vi "Save info to spreadsheet.vi"(8 "Cell Settings Array":T1(array[cluster])=[{"Cell Position"=1, "Cell Label"="", "Pixel to measure"=0, "Area (cm^2)"=0.126, "Variable"="", "Variable value"="", "Scan settings in queue"=0}, {"Cell Position"=2, "Cell Label"="", "Pixel to measure"=0, "Area (cm^2)"=0.126, "Variable"="", "Variable value"="", "Scan settings in queue"=0}, {"Cell Position"=3, "Cell Label"="", "Pixel to measure"=0, "Area (cm^2)"=0.126, "Variable"="", "Variable value"="", "Scan settings in queue"=0}, {"Cell Position"=4, "Cell Label"="", "Pixel to measure"=0, "Area (cm^2)"=0.126, "Variable"="", "Variable value"="", "Scan settings in queue"=0}, {"Cell Position"=5, "Cell Label"="", "Pixel to measure"=0, "Area (cm^2)"=0.126, "Variable"="", "Variable value"="", "Scan settings in queue"=0}, {"Cell Position"=6, "Cell Label"="", "Pixel to measure"=0, "Area (cm^2)"=0.126, "Variable"="", "Variable value"="", "Scan settings in queue"=0}, {"Cell Position"=7, "Cell Label"="", "Pixel to measure"=0, "Area (cm^2)"=0.126, "Variable"="", "Variable value"="", "Scan settings in queue"=0}, {"Cell Position"=8, "Cell Label"="", "Pixel to measure"=0, "Area (cm^2)"=0.126, "Variable"="", "Variable value"="", "Scan settings in queue"=0}, {"Cell Position"=9, "Cell Label"="", "Pixel to measure"=0, "Area (cm^2)"=0.126, "Variable"="", "Variable value"="", "Scan settings in queue"=0}, {"Cell Position"=10, "Cell Label"="", "Pixel to measure"=0, "Area (cm^2)"=0.126, "Variable"="", "Variable value"="", "Scan settings in queue"=0}, {"Cell Position"=11, "Cell Label"="", "Pixel to measure"=0, "Area (cm^2)"=0.126, "Variable"="", "Variable value"="", "Scan settings in queue"=0}, {"Cell Position"=12, "Cell Label"="", "Pixel to measure"=0, "Area (cm^2)"=0.126, "Variable"="", "Variable value"="", "Scan settings in queue"=0}, {"Cell Position"=13, "Cell Label"="", "Pixel to measure"=0, "Area (cm^2)"=0.126, "Variable"="", "Variable value"="", "Scan settings in queue"=0}, {"Cell Position"=14, "Cell Label"="", "Pixel to measure"=0, "Area (cm^2)"=0.126, "Variable"="", "Variable value"="", "Scan settings in queue"=0}, {"Cell Position"=15, "Cell Label"="", "Pixel to measure"=0, "Area (cm^2)"=0.126, "Variable"="", "Variable value"="", "Scan settings in queue"=0}, {"Cell Position"=16, "Cell Label"="", "Pixel to measure"=0, "Area (cm^2)"=0.126, "Variable"="", "Variable value"="", "Scan settings in queue"=0}] {"Pixel to measure" items=["All", "1", "2", "3", "4", "5", "6", "7", "8"]}) -> ()   [LabVIEW 2011]
uses:
  <vilib>/Utility/file.llb/Write To Spreadsheet File (string).vi
panel:
  out "error out":errorcluster
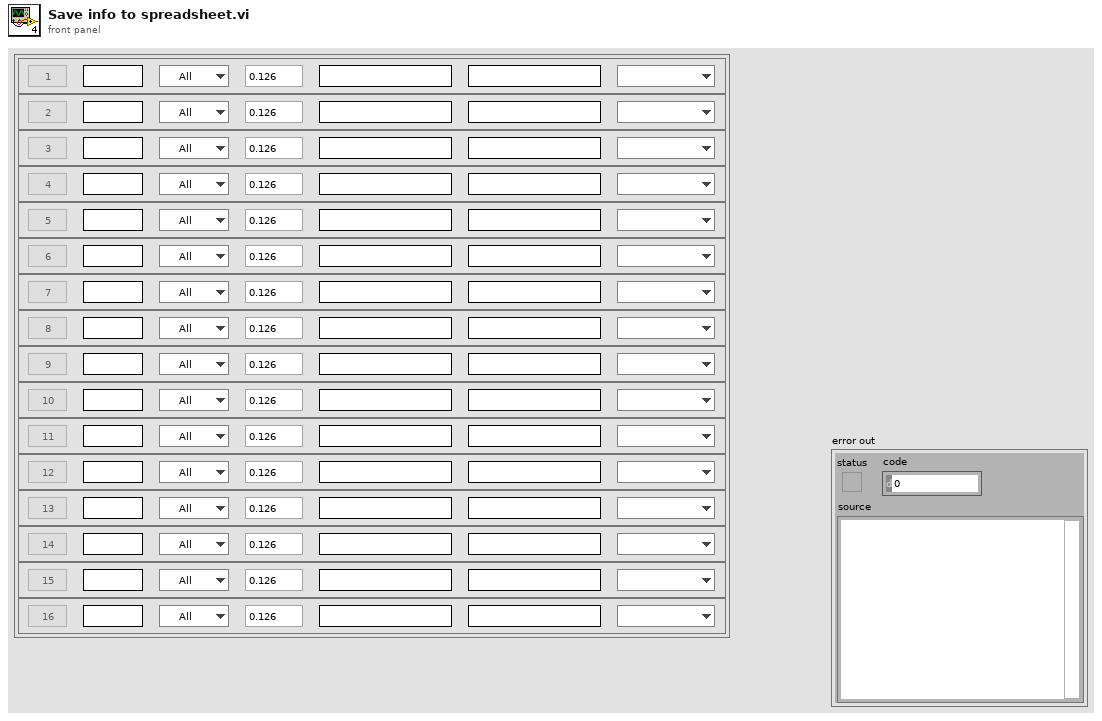
[diagram p1: front panel]
types:
  T1 = cluster{"Cell Position":i32, "Cell Label":string, "Pixel to measure":u16, "Area (cm^2)":dbl, "Variable":string, "Variable value":string, "Scan settings in queue":u16}[]
  T2 = enum16{"open", "replace", "create", "open or create", "replace or create", "replace or create with confirmation"}
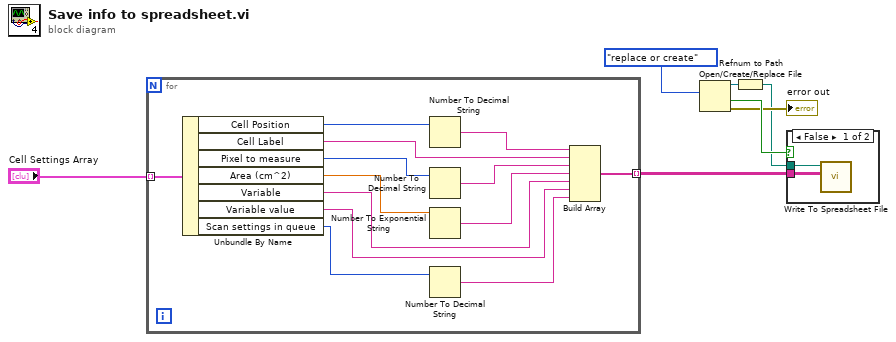
[diagram p0: block diagram]
diagram:
  n1 = for {
    tunnel: "Cell Settings Array" -> [w20] mode=indexing
    tunnel: [w8] -> w6 mode=indexing
    n2 = Unbundle By Name(w20) -> ("Cell Position"=w19:i32, "Cell Label"=w14:string, "Pixel to measure"=w18:u16, "Area (cm^2)"=w17:dbl, "Variable"=w11:string, "Variable value"=w10:string, "Scan settings in queue"=w16:u16)
    n3 = Number To Decimal String(number=w19) -> (decimal integer string=w15:string)  [unwired: 1 in]
    n4 = Number To Decimal String(number=w18) -> (decimal integer string=w13:string)  [unwired: 1 in]
    n5 = Number To Exponential String(number=w17) -> (E-format string=w12:string)  [unwired: 3 in]
    n6 = Number To Decimal String(number=w16) -> (decimal integer string=w9:string)  [unwired: 1 in]
    n7 = Build Array(w15, w14, w13, w12, w11, w10, w9) -> (w8:string[])
  }
  n8 = Open/Create/Replace File(operation (0:open)=T2."replace or create") -> (refnum out=w2:refnum<file>, cancelled=w4:bool, error out=→"error out":errorcluster)  [unwired: 5 in]
  n9 = Refnum to Path(1:w2) -> (0:w1:path)
  n10 = case shown="False" w4 {
    tunnel: w6 -> [w22 _]
    tunnel: w1 -> [w21 _]
    frame False {
      n11 = call-poly <vilib>:"Write To Spreadsheet File.vi"("2D data"=w22, "file path (dialog if empty)"=w21) -> ()  [unwired: 6 in, 1 out]
    }
    frame True {
    }
  }
